vi "Cleanup Session.vi"(8 "error in":errorcluster, 11 "Plugin in":refnum<class "PXIe-4113 DC Power Supply NI-DCPower Runtime Plugin PowerSupply.lvclass">) -> (0 "error out":errorcluster, 3 "Plugin out":refnum<class "PXIe-4113 DC Power Supply NI-DCPower Runtime Plugin PowerSupply.lvclass">)   [LabVIEW 2026, in "PXIe-4113 DC Power Supply NI-DCPower Runtime Plugin PowerSupply.lvlib" / "PXIe-4113 DC Power Supply NI-DCPower Runtime Plugin PowerSupply.lvclass"]
uses:
  PXIe-4113 DC Power Supply NI-DCPower Runtime Plugin PowerSupply.lvclass
  PXIe-4113 DC Power Supply NI-DCPower Runtime Plugin PowerSupply.lvclass/PXIe-4113 DC Power Supply NI-DCPower Runtime Plugin PowerSupply.ctl
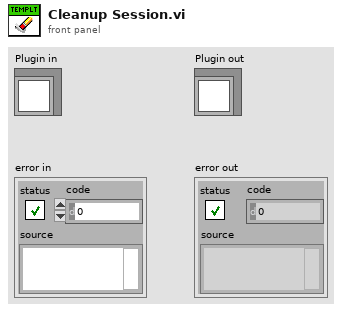
[diagram p1: front panel]
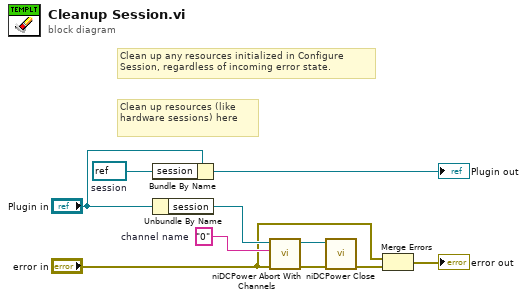
[diagram p0: block diagram]
diagram:
  w6 = refnum<k15> refnum  # session
  w9 = "0"  # channel name
  # "Clean up resources (like hardware sessions) here"
  # "Clean up any resources initialized in Configure Session, regardless of incoming error state."
  n1 = Bundle By Name(cluster="Plugin in", "session"=w6) -> (→"Plugin out":refnum<class "PXIe-4113 DC Power Supply NI-DCPower Runtime Plugin PowerSupply.lvclass">)
  n2 = Unbundle By Name("Plugin in") -> ("session"=w10:refnum<k15>)
  n3 = call <instrlib>:"niDCPower Abort With Channels.vi"("error in (no error)"="error in", "channel name"=w9, "instrument handle"=w10) -> ("error out"=w7:errorcluster, "instrument handle out"=w8:refnum<k15>)  [unwired: 7 in]
  n4 = call <instrlib>:"niDCPower Close.vi"("error in (no error)"=w7, "instrument handle"=w8) -> ("error out"=w2:errorcluster)  [unwired: 9 in]
  n5 = Merge Errors("error in", w2) -> (→"error out":errorcluster)
